vi "Actor Core.vi"(8 "error in":errorcluster, 11 "Server in":refnum<class "Server.lvclass">) -> (0 "error out":errorcluster, 3 "Actor out":refnum<class "Actor.lvclass">)   [LabVIEW 2018, in "Server.lvlib" / "Server.lvclass"]
doc: "(<B>Filename</B>: Actor Framework.lvlib:Actor.lvclass:Actor Core.vi)\n\nReceives messages to the actor, reacts to them, and initiates any error handling that may shut the actor down.\n\nDescendant classes may override this VI to append parallel tasks for the actor to complete while it handles messages. Overrides use the Call Parent Method node."
uses:
  Server.lvclass
  C:/Program Files (x86)/National Instruments/LabVIEW 2018/vi.lib/ActorFramework/Actor/Actor.lvclass
  <vilib>/ActorFramework/Actor/Actor.lvclass
  <vilib>/ActorFramework/Actor/Actor.lvclass/Actor.ctl
  <vilib>/ActorFramework/Message Enqueuer/Message Enqueuer.lvclass/Message Enqueuer.ctl
  Server.lvclass/Server.ctl
  <vilib>/ActorFramework/Message Enqueuer/Init from Existing Queue.vi
  <vilib>/ActorFramework/Message Enqueuer/Enqueue.vi
  Server Messages/Send Global Chat Msg/Send Global Chat Msg.lvclass
  C:/Program Files (x86)/National Instruments/LabVIEW 2018/vi.lib/ActorFramework/Message/Message.lvclass
  <vilib>/ActorFramework/Stop Msg/Stop Msg.lvclass
  Server Messages/Launch New Chat Window Msg/Launch New Chat Window Msg.lvclass
  <vilib>/ActorFramework/Message Priority Queue/Priority Enqueue.vi
  <vilib>/ActorFramework/Message Enqueuer/Message Enqueuer.lvclass
panel:
  in  "Send Chat":bool
  in  "Message":string
  in  "Launch Chat Window":bool
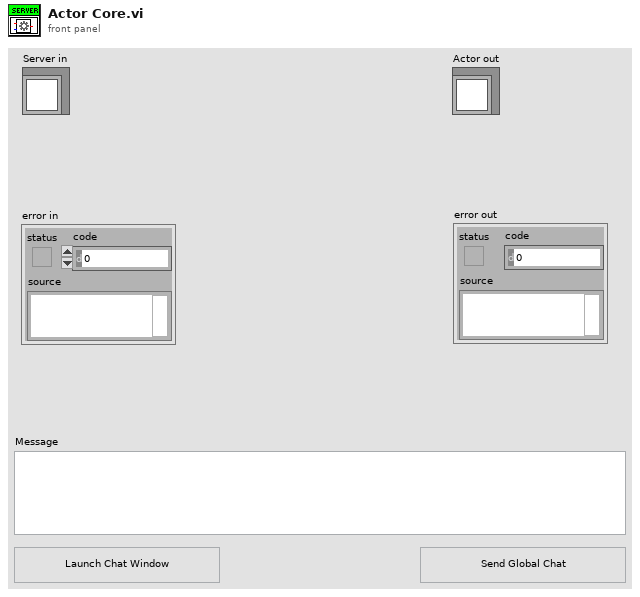
[diagram p1: front panel]
types:
  T1 = enum32{"Invalid", "Standard", "Closed", "Hidden", "Minimized", "Maximized"}
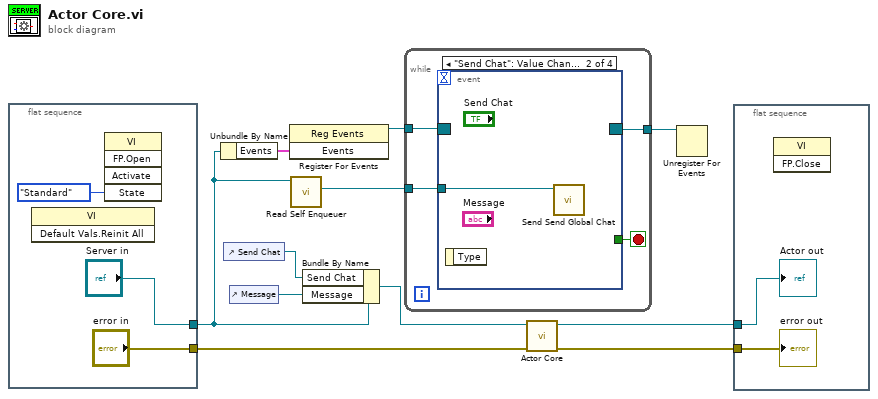
[diagram p0: block diagram]
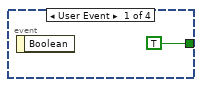
[diagram p2: hidden frame]
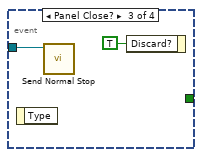
[diagram p3: hidden frame]
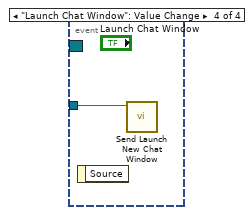
[diagram p4: hidden frame]
diagram:
  n1 = flat-sequence {
    tunnel: ["error in"] -> w1
    tunnel: ["Server in"] -> w5
    frame #0 {
      n2 = invoke class="VI" method="Default Vals.Reinit All"() -> ()  [unwired: 3 in, 3 out]
      n3 = invoke class="VI" method="FP.Open"("State"=T1."Standard") -> ()  [unwired: 4 in, 5 out]
    }
  }
  n4 = Unbundle By Name(w5) -> ("Events"=w9:cluster{"Stop":refnum<user-event>})
  n5 = control-ref of="Send Chat"() -> (w3:refnum<vi>)
  n6 = control-ref of="Message"() -> (w4:refnum<vi>)
  n7 = register-events(w9) -> (reference out=w8:refnum<event-registration>)  [unwired: 2 in, 1 out]
  n8 = call <vilib>:"Read Self Enqueuer.vi"("Actor"=w5) -> ("Self Enqueuer"=w6:refnum<class "Message Enqueuer.lvclass">)  [unwired: 10 in]
  n9 = Bundle By Name(cluster=w5, "Send Chat"=w3, "Message"=w4) -> (w2:refnum<class "Server.lvclass">)
  n10 = while {
    tunnel: w8 -> [w18]
    tunnel: [w16] -> w7
    tunnel: w6 -> [w15]
    stop <- w17 stop-if-true
    n11 = event shown="[1] \"Send Chat\": Value Change" {
      selector: w18 -> [_ _ _ _]
      dyn-events: [_ _ _ _] -> w16
      timeout: _ -> [_ _ _ _]
      tunnel: [TRUE _ _ _] -> w17
      tunnel: w15 -> [_ w20 w21 w23]
      event User Event {
        n12 = event-data() -> ()  [unwired: 1 in, 1 out]
      }
      event "Send Chat": Value Change {
        n13 = event-data() -> ()  [unwired: 1 in, 1 out]
        n14 = call "Send Send Global Chat.vi"("Message Enqueuer"=w20) -> ()  [unwired: 9 in, 2 out]
      }
      event Panel Close? {
        n15 = event-data() -> ()  [unwired: 1 in, 1 out]
        n16 = call <vilib>:"Send Normal Stop.vi"("Message Enqueuer"=w21) -> ()  [unwired: 10 in, 1 out]
        n17 = event-data("Discard?"=TRUE) -> ()  [unwired: 1 in, 1 out]
      }
      event "Launch Chat Window": Value Change {
        n18 = event-data() -> ()  [unwired: 1 in, 1 out]
        n19 = call "Send Launch New Chat Window.vi"("Message Enqueuer"=w23) -> ()  [unwired: 9 in, 2 out]
      }
    }
  }
  n20 = call-parent "Actor Core.vi"("error in"=w1, "Actor in"=w2) -> ("error out"=w11:errorcluster, "Actor out"=w10:refnum<class "Actor.lvclass">)  [unwired: 8 in]
  n21 = Unregister For Events(event registration refnum=w7) -> ()  [unwired: 1 in, 1 out]
  n22 = flat-sequence {
    tunnel: w11 -> [w25]
    tunnel: w10 -> [w24]
    frame #0 {
      n23 = invoke class="VI" method="FP.Close"() -> ()  [unwired: 3 in, 3 out]
      "error out" <- w25
      "Actor out" <- w24
    }
  }
